vi "ExTestDevInput.vi"() -> ()   [LabVIEW 2010]
panel:
  out "Device IO direction":u32
  in  "Device Address":u32
  in  "stop":bool
  out "Device Value":dbl format="%.2f"
  out "Device Bit Depth":u32
  out "Device Type":u32
  out "error out":errorcluster
  in  "error in (no error)":errorcluster
  # "ExTestDevInput\nThis example shows how to read from\nthe TTL lines on the camera. This \nprogram will  loop until stop button is\npressed, it will continously read the \nttl port in the loop\nNote: not all camera systems have this\nfeature."
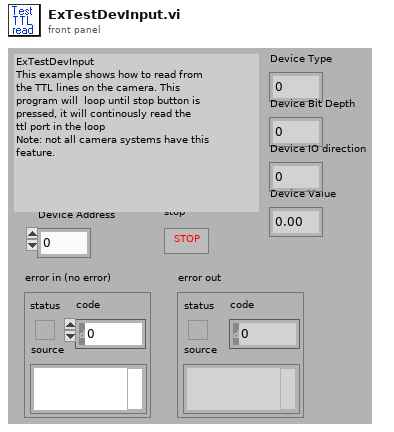
[diagram p1: front panel]
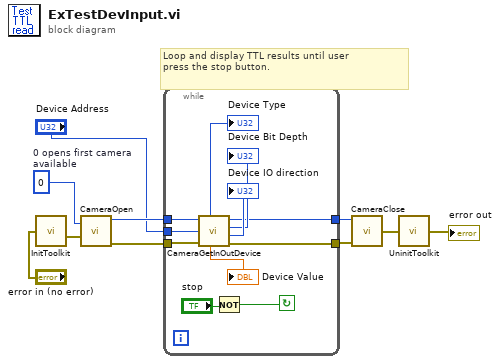
[diagram p0: block diagram]
diagram:
  w2 = 0  # 0 opens first camera  available
  # "Loop and display TTL results until user\npress the stop button."
  n1 = call <userlib>:"InitToolkit.vi"("error in"="error in (no error)") -> ("error out"=w7:errorcluster)
  n2 = call <userlib>:"CameraOpen.vi"("error in"=w7, "Camera Device ID"=w2) -> ("error out"=w5:errorcluster, "Camera Handle"=w6:u32)
  n3 = while {
    tunnel: w6 -> [w19]
    tunnel: w5 -> [w18]
    tunnel: [w17] -> w4
    tunnel: "Device Address" -> [w16]
    tunnel: [w12] -> w1
    stop <- w21 continue-if-true
    n4 = call <userlib>:"CameraGetInOutDevice.vi"("Camera Handle"=w19, "Device Address"=w16, "error in"=w18) -> ("Device type"=→"Device Type":u32, "Input from device"=→"Device Value":dbl, "Camera Handle"=w12:u32, "Device Bit depth"=→"Device Bit Depth":u32, "Device IO direction"=→"Device IO direction":u32, "error out"=w17:errorcluster)
    n5 = Not(x="stop") -> (.not. x?=w21:bool)
  }
  n6 = call <userlib>:"CameraClose.vi"("error in"=w4, "Camera Handle"=w1) -> ("error out"=w8:errorcluster)
  n7 = call <userlib>:"UninitToolkit.vi"("error in"=w8) -> ("error out"=→"error out":errorcluster)
